vi "lib Parse Numeric Range String to array.vi"(8 "error in (no error)":errorcluster, 11 "Masses":string caption="Range String") -> (0 "error out":errorcluster, 3 "Array":i32[](array[numeric]))   [LabVIEW 2014]
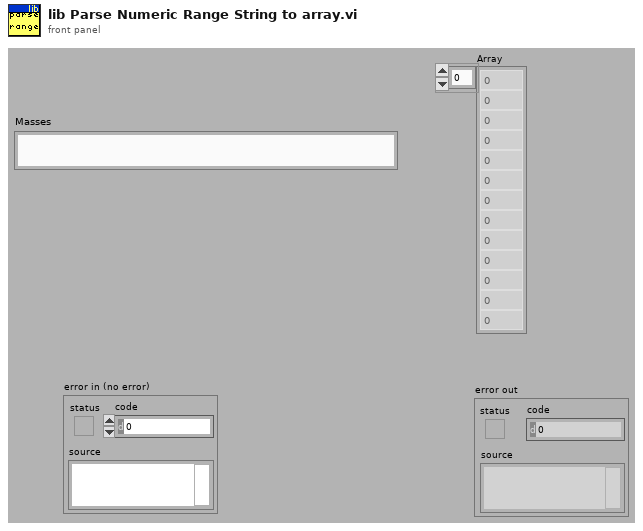
[diagram p1: front panel]
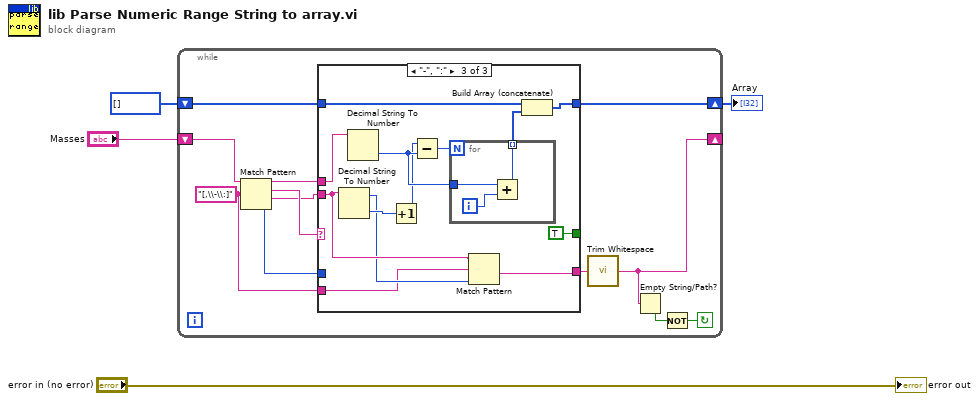
[diagram p0: block diagram]
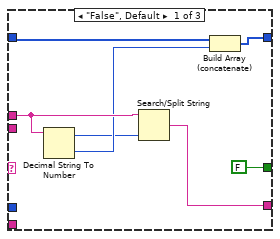
[diagram p2: hidden frame]
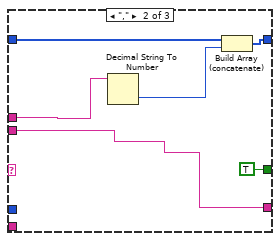
[diagram p3: hidden frame]
diagram:
  n1 = while {
    shift-right: [w9] -> _
    shift-left: "Masses" -> [w16]
    shift-right: [w13] -> w1
    shift-left: i32[] [] -> [w14]
    stop <- w11 continue-if-true
    w5 = "[,\\-\\:]" ("regular expression")
    n2 = Match Pattern(string=w16, regular expression=w5) -> (before substring=w15:string, match substring=w7:string, after substring=w6:string, offset past match=w8:i32)  [unwired: 1 in]
    n3 = case shown="\"-\", \":\"" w7 {
      tunnel: w15 -> [w20 w25 w34]
      tunnel: w14 -> [w23 w29 w37]
      tunnel: [w22 w28 w36] -> w13
      tunnel: [FALSE TRUE TRUE] -> _
      tunnel: [w18 w24 w30] -> w12
      tunnel: w8 -> [_ _ _]
      tunnel: w6 -> [_ w24 w33]
      tunnel: w5 -> [_ _ w31]
      frame "False", Default {
        n4 = Decimal String To Number(string=w20) -> (offset past number=w17:i32, number=w19:i32)  [unwired: 2 in]
        n5 = Search/Split String(string=w20, offset (0)=w17) -> (match + rest of string=w18:string)  [unwired: 1 in, 2 out]
        n6 = Build Array (concatenate)(w23, w19) -> (w22:i32[])
      }
      frame "," {
        n7 = Decimal String To Number(string=w25) -> (number=w26:i32)  [unwired: 2 in, 1 out]
        n8 = Build Array (concatenate)(w29, w26) -> (w28:i32[])
      }
      frame "-", ":" {
        n9 = Decimal String To Number(string=w33) -> (offset past number=w32:i32, number=w41:i32)  [unwired: 2 in]
        n10 = Decimal String To Number(string=w34) -> (number=w40:i32)  [unwired: 2 in, 1 out]
        n11 = Increment(x=w41) -> (x+1=w39:i32)
        n12 = Subtract(x=w39, y=w40) -> (x-y=w42:i32)
        n13 = for {
          N: w42 -> [_]
          tunnel: w40 -> [w44]
          tunnel: [w43] -> w38 mode=indexing
          i -> [w45]
          n14 = Add(x=w44, y=w45) -> (x+y=w43:i32)
        }
        n15 = Match Pattern(string=w33, regular expression=w31, offset (0)=w32) -> (after substring=w30:string)  [unwired: 3 out]
        n16 = Build Array (concatenate)(w37, w38) -> (w36:i32[])
      }
    }
    n17 = call <vilib>:"Trim Whitespace.vi"("string"=w12) -> ("trimmed string"=w9:string)  [unwired: 1 in]
    n18 = Empty String/Path?(string/path=w9) -> (empty?=w10:bool)
    n19 = Not(x=w10) -> (.not. x?=w11:bool)
  }
  "Array" <- w1
  "error out" <- "error in (no error)"
